vi "final project.vi"() -> ()   [LabVIEW 2014]
uses:
  <vilib>/Utility/file.llb/Read From Spreadsheet File (DBL).vi
  <vilib>/Utility/file.llb/Write To Spreadsheet File (DBL).vi
panel:
  out "發電機開啟":bool
  out "馬達所需能量(W)":dbl(graph)
  out "電池shut down SOC(%)":dbl
  out "電量SOC變化(%)":dbl
  out "剩餘油量(L)":dbl
  out "電量SOC變化(%)":dbl(graph)
  out "油量變化":dbl(graph)
  out "電量需求發電機開啟":bool
  in  "路徑模擬初始值設定":T1={"發電機開啟SOC(%)"="50", "發電機關閉SOC(%)"="80", "電池初始SOC(%) "="100", "電池shut down SOC(%) "="20", "油箱容量(L)"="3"}
  out "引擎熱效率(%)":dbl
  out "發電機效率(%)":dbl
  out "發電機功率(kW)":dbl
  out "電池效率(%)":dbl
  out "功率需求發電機開啟":bool
  out "電池容量(kWh)":dbl
  out "電池最大放電C-rate":dbl
  out "馬達驅動器效率(%)":dbl
  out "馬達效率(%)":dbl
  out "馬達輸出轉速(rpm)":dbl(graph)
  out "馬達輸出扭矩(Nm)":dbl(graph)
  out "車輛目前速度(kph)":dbl(graph)
  in  "停止模擬":bool
  out "馬達輸出轉速":dbl
  out "目標路徑WMTC":dbl(graph)
  out "輪胎半徑(mm)":dbl
  in  "模擬路徑":path=path "E:/碩士班/碩二下課堂/虛擬儀控之設計與應用/WMTC1-2.lvm"
  out "傳動效率(%)":dbl
  out "馬達最大轉速(rpm)":dbl
  out "馬達最大扭矩(Nm)":dbl
  out "馬達功率(kW)":dbl
  out "傳動比":dbl
  in  "開始模擬":bool
  in  "動力系統元件規格":T2={"馬達功率(kW)"="8", "馬達最大扭矩(Nm)"="30", "馬達最大轉速(rpm)"="10000", "發電機功率(kW)"="4", "發電機效率(%)"="90", "引擎熱效率(%)"="20", "電池容量(kWh)"="2", "電池效率(%)"="90", "電池最大放電C-rate"="4", "傳動比"="9", "傳動效率(%)"="85", "馬達效率(%)"="90", "MCU效率(%)"="95"}
  in  "車輛參數設定":T3={"車重(kg)"="150", "人重(kg)"="75", "人數"="1", "CdA (m^2)"="0.37", "滾阻係數"="0.0256", "重力加速度(m/s^2)"="9.81", "空氣密度(kg/m^3)"="1.225", "輪胎半徑(mm)"="0.242"}
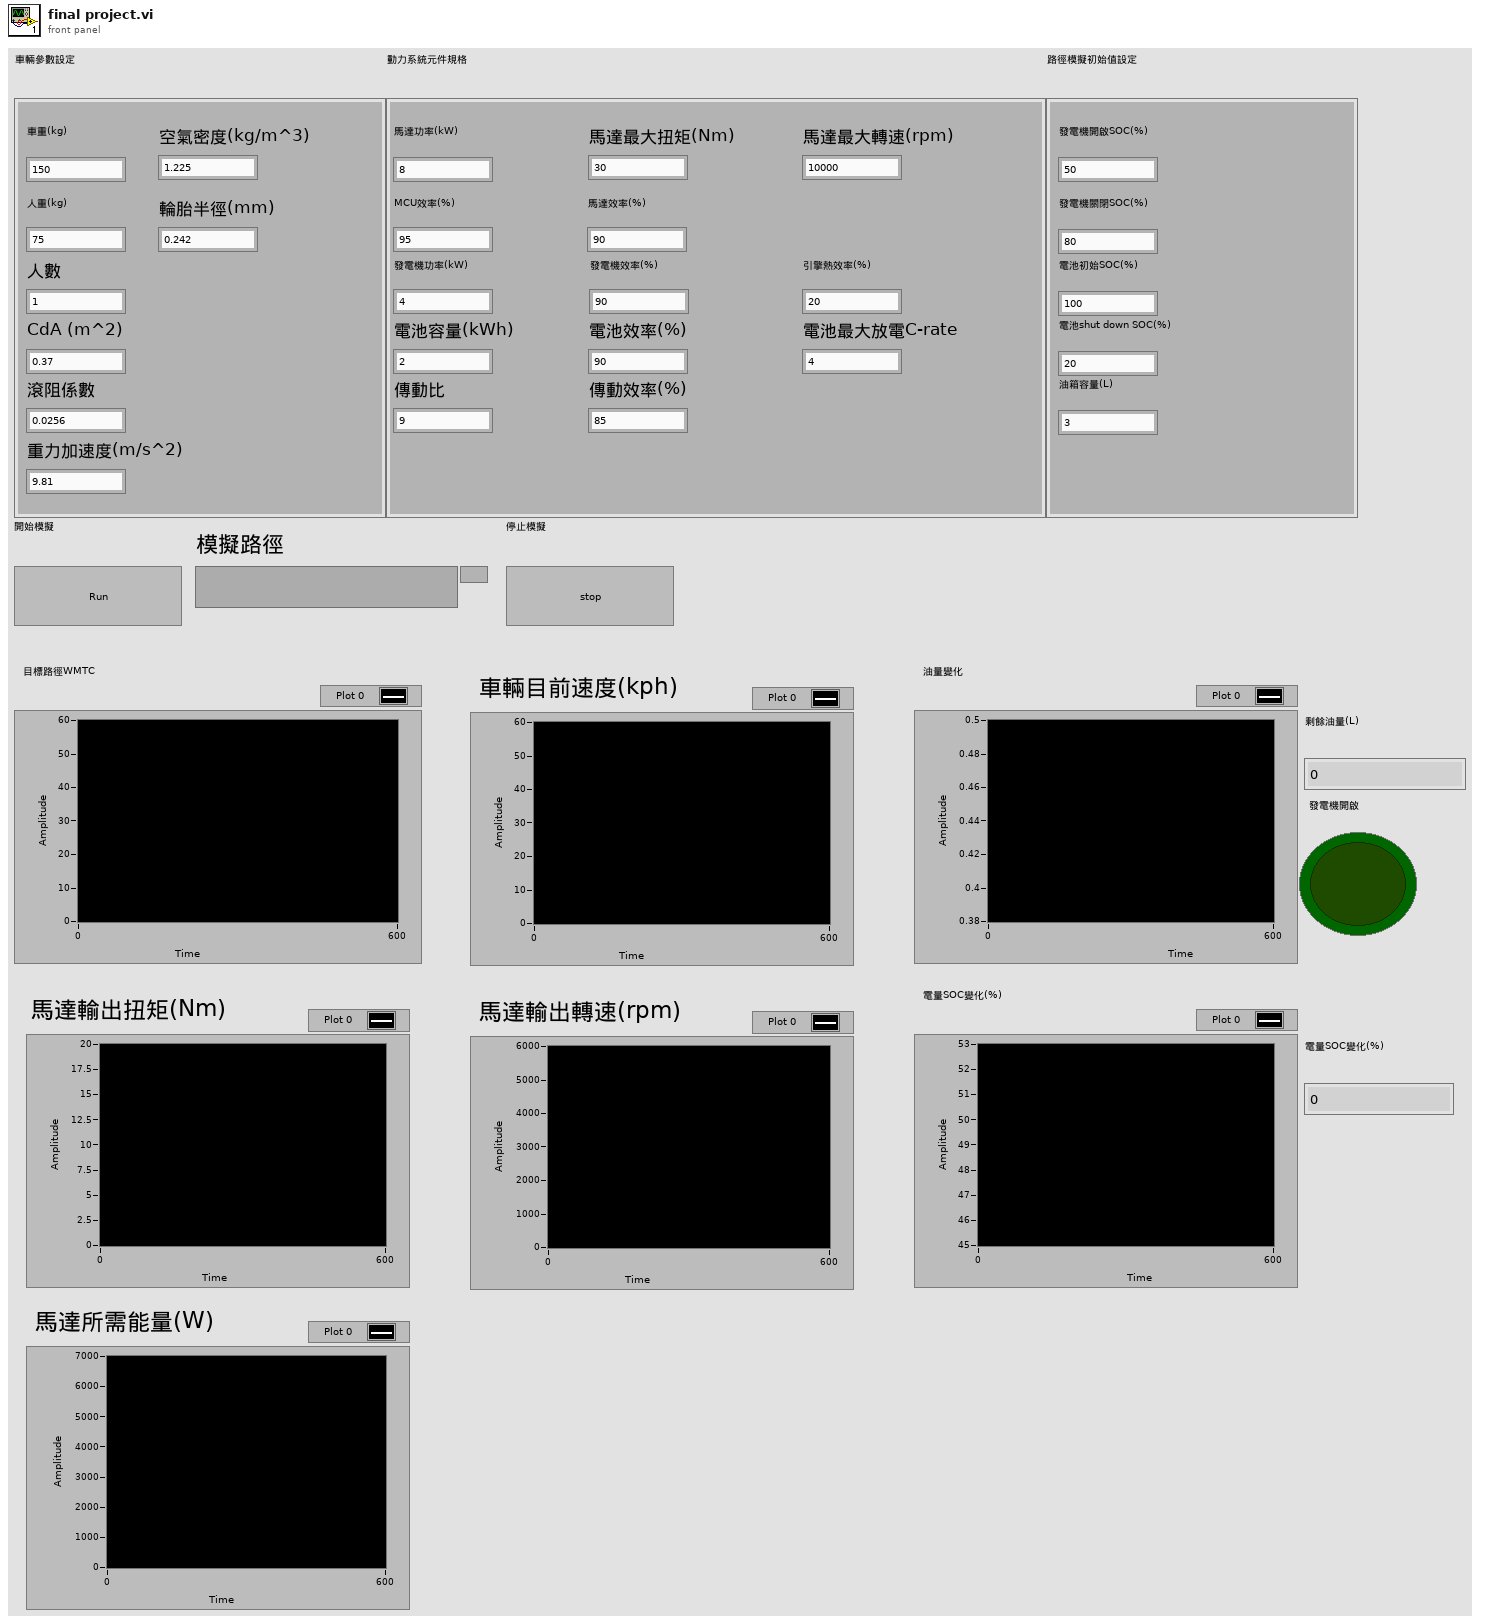
[diagram p1: front panel]
types:
  T1 = cluster{"發電機開啟SOC(%)":string, "發電機關閉SOC(%)":string, "電池初始SOC(%) ":string, "電池shut down SOC(%) ":string, "油箱容量(L)":string}
  T2 = cluster{"馬達功率(kW)":string, "馬達最大扭矩(Nm)":string, "馬達最大轉速(rpm)":string, "發電機功率(kW)":string, "發電機效率(%)":string, "引擎熱效率(%)":string, "電池容量(kWh)":string, "電池效率(%)":string, "電池最大放電C-rate":string, "傳動比":string, "傳動效率(%)":string, "馬達效率(%)":string, "MCU效率(%)":string}
  T3 = cluster{"車重(kg)":string, "人重(kg)":string, "人數":string, "CdA (m^2)":string, "滾阻係數":string, "重力加速度(m/s^2)":string, "空氣密度(kg/m^3)":string, "輪胎半徑(mm)":string}
  T4 = cluster{"馬達功率(kW)":dbl, "馬達最大扭矩(Nm)":dbl, "馬達最大轉速(rpm)":dbl, "發電機功率(kW)":dbl, "發電機效率(%)":dbl, "引擎熱效率(%)":dbl, "電池容量(kWh)":dbl, "電池效率(%)":dbl, "電池最大放電C-rate":dbl, "傳動比":dbl, "傳動效率(%)":dbl, "馬達效率(%)":dbl, "MCU效率(%)":dbl}
  T5 = cluster{"發電機開啟SOC(%)":dbl, "發電機關閉SOC(%)":dbl, "電池初始SOC(%) ":dbl, "電池shut down SOC(%) ":dbl, "油箱容量(L)":dbl}
  T6 = cluster{"車重(kg)":dbl, "人重(kg)":dbl, "人數":dbl, "CdA (m^2)":dbl, "滾阻係數":dbl, "重力加速度(m/s^2)":dbl, "空氣密度(kg/m^3)":dbl, "輪胎半徑(mm)":dbl}
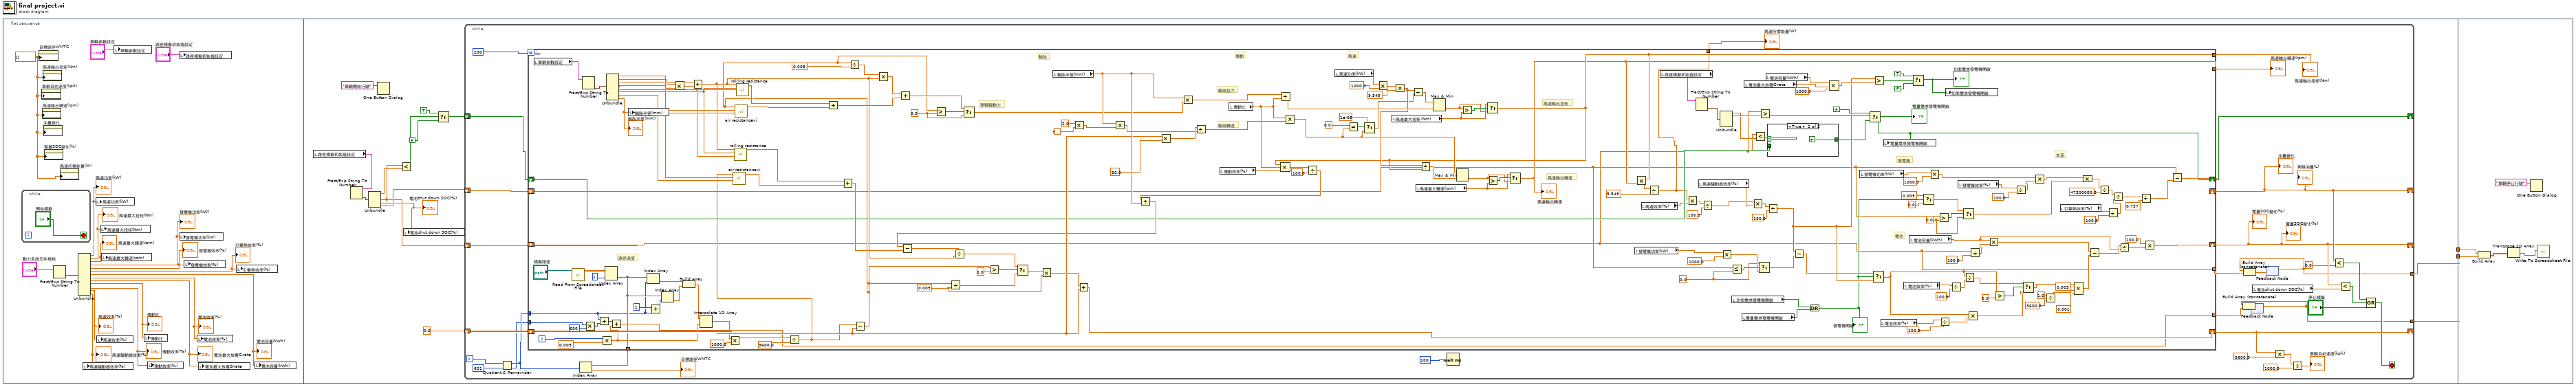
[diagram p0: block diagram]
diagram:
  n1 = flat-sequence {
    tunnel: [w23] -> w2
    tunnel: [w22] -> w1
    tunnel: w2 -> [w259]
    tunnel: w1 -> [w258]
    frame #0 {
      w3 = dbl[] [] ("History Data")
      n2 = while {
        stop <- "開始模擬" stop-if-true
      }
      n3 = property on="目標路徑WMTC" class="WFChart (strict)"("History Data"=w3) -> ()  [unwired: 2 in, 2 out]
      n4 = property on="車輛目前速度(kph)" class="WFChart (strict)"("History Data"=w3) -> ()  [unwired: 2 in, 2 out]
      n5 = property on="馬達輸出轉速(rpm)" class="WFChart (strict)"("History Data"=w3) -> ()  [unwired: 2 in, 2 out]
      n6 = property on="馬達輸出扭矩(Nm)" class="WFChart (strict)"("History Data"=w3) -> ()  [unwired: 2 in, 2 out]
      n7 = property on="油量變化" class="WFChart (strict)"("History Data"=w3) -> ()  [unwired: 2 in, 2 out]
      n8 = property on="電量SOC變化(%)" class="WFChart (strict)"("History Data"=w3) -> ()  [unwired: 2 in, 2 out]
      n9 = Fract/Exp String To Number(string="動力系統元件規格") -> (number=w19:T4)  [unwired: 3 in, 1 out]
      n10 = property on="馬達所需能量(W)" class="WFChart (strict)"("History Data"=w3) -> ()  [unwired: 2 in, 2 out]
      n11 = Unbundle(w19) -> ("馬達功率(kW)"=w17:dbl, "馬達最大扭矩(Nm)"=w16:dbl, "馬達最大轉速(rpm)"=w15:dbl, "發電機功率(kW)"=w7:dbl, "發電機效率(%)"=w6:dbl, "引擎熱效率(%)"=w5:dbl, "電池容量(kWh)"=w9:dbl, "電池效率(%)"=w8:dbl, "電池最大放電C-rate"=w10:dbl, "傳動比"=w18:dbl, "傳動效率(%)"=w14:dbl, "馬達效率(%)"=w12:dbl, "MCU效率(%)"=w11:dbl)
      "傳動比" <- w18
      "馬達功率(kW)" <- w17
      "馬達最大扭矩(Nm)" <- w16
      "馬達最大轉速(rpm)" <- w15
      "傳動效率(%)" <- w14
      "馬達效率(%)" <- w12
      "馬達驅動器效率(%)" <- w11
      "電池最大放電C-rate" <- w10
      "電池容量(kWh)" <- w9
      "電池效率(%)" <- w8
      "發電機功率(kW)" <- w7
      "發電機效率(%)" <- w6
      "引擎熱效率(%)" <- w5
      n12 = local write "馬達驅動器效率(%)"(w11) -> ()
      n13 = local write "馬達功率(kW)"(w17) -> ()
      n14 = local write "馬達效率(%)"(w12) -> ()
      n15 = local write "馬達最大扭矩(Nm)"(w16) -> ()
      n16 = local write "馬達最大轉速(rpm)"(w15) -> ()
      n17 = local write "車輛參數設定"("車輛參數設定") -> ()
      n18 = local write "傳動比"(w18) -> ()
      n19 = local write "傳動效率(%)"(w14) -> ()
      n20 = local write "路徑模擬初始值設定"("路徑模擬初始值設定") -> ()
      n21 = local write "發電機功率(kW)"(w7) -> ()
      n22 = local write "發電機效率(%)"(w6) -> ()
      n23 = local write "電池效率(%)"(w8) -> ()
      n24 = local write "電池最大放電C-rate"(w10) -> ()
      n25 = local write "引擎熱效率(%)"(w5) -> ()
      n26 = local write "電池容量(kWh)"(w9) -> ()
    }
    frame #1 {
      n27 = local read "路徑模擬初始值設定"() -> (w34:T1)
      n28 = Fract/Exp String To Number(string=w34) -> (number=w33:T5)  [unwired: 3 in, 1 out]
      n29 = Unbundle(w33) -> ("發電機開啟SOC(%)"=w30:dbl, "電池初始SOC(%)"=w29:dbl, "電池shut down SOC(%)"=w32:dbl, "油箱容量(L)"=w31:dbl)  [unwired: 1 out]
      "電池shut down SOC(%)" <- w32
      n30 = One Button Dialog(message="車輛開始行駛") -> ()  [unwired: 1 in, 1 out]
      n31 = Less?(x=w29, y=w30) -> (x < y?=w26:bool)
      n32 = local write "電池shut down SOC(%)"(w32) -> ()
      n33 = Select(t=TRUE, s=w26, f=FALSE) -> (s? t:f=w25:bool)
      n34 = while {
        shift-right: [w61] -> _
        shift-left: 0.0 ("y") -> [w69]
        shift-right: [w53] -> _
        shift-left: w31 -> [w55]
        shift-right: [w52] -> _
        shift-left: w29 -> [w54]
        shift-right: [w44] -> _
        shift-left: w25 -> [w45]
        tunnel: [w40] -> w22
        tunnel: [w37] -> w23
        i -> [w66]
        stop <- w48 stop-if-true
        n35 = Quotient & Remainder(x=w66, y=601) -> (x-y*floor(x/y)=w59:i32, floor(x/y)=w36:i32)
        n36 = for {
          N: 200 -> [_]
          shift-right: [w182] -> w61
          shift-left: w69 -> [w186]
          tunnel: w59 -> [w72]
          tunnel: [w83] -> w60
          tunnel: [w174] -> w57
          tunnel: [w173] -> w56
          shift-right: [w132] -> w52
          shift-left: w54 -> [w78]
          shift-right: [w109] -> w53
          shift-left: w55 -> [w96]
          shift-right: [w85] -> w44
          shift-left: w45 -> [w86]
          tunnel: [w79] -> w43
          tunnel: [w78] -> w42 mode=indexing
          tunnel: [w75] -> w39 mode=indexing
          tunnel: w36 -> [w74]
          i -> [w175]
          w87 = 0.0 ("y")
          w98 = 0.0 ("y")
          w188 = 0.005 ("y")
          w201 = 0.0 ("y")
          # "ま篮"
          # "發電機"
          # "電池"
          # "馬達"
          # "輪胎"
          # "傳動"
          # "車輛驅動力"
          # "路徑速度"
          # "馬達輸出轉速"
          # "馬達輸出扭矩"
          # "輪端轉速"
          # "輪端扭力"
          n37 = local read "車輛參數設定"() -> (w217:T3)
          n38 = call-poly <vilib>:"Read From Spreadsheet File.vi"("file path (dialog if empty)"="模擬路徑") -> ("all rows"=w219:dbl[][])  [unwired: 6 in, 4 out]
          n39 = Fract/Exp String To Number(string=w217) -> (number=w218:T6)  [unwired: 3 in, 1 out]
          n40 = Multiply(x=w74, y=600) -> (x*y=w73:i32)
          n41 = Add(x=w72, y=w73) -> (x+y=w71:i32)
          n42 = Multiply(x=w175, y=0.005) -> (x*y=w76:dbl)
          n43 = Index Array(array=w219, index (col)=1 ("index (row)")) -> (element=w83:dbl[])  [unwired: 1 in]
          n44 = Unbundle(w218) -> ("車重(kg)"=w216:dbl, "人重(kg)"=w214:dbl, "人數"=w215:dbl, "CdA (m^2)"=w212:dbl, "滾阻係數"=w211:dbl, "重力加速度(m/s^2)"=w210:dbl, "空氣密度(kg/m^3)"=w209:dbl, "輪胎半徑(mm)"=w208:dbl)
          "輪胎半徑(mm)" <- w208
          n45 = Add(x=w71, y=w76) -> (x+y=w75:dbl)
          n46 = local write "輪胎半徑(mm)"(w208) -> ()
          n47 = Index Array(array=w83, index=w72) -> (element=w178:dbl)
          n48 = Add(x=1, y=w72) -> (x+y=w180:i32)
          n49 = Index Array(array=w83, index=w180) -> (element=w177:dbl)
          n50 = Multiply(x=w214, y=w215) -> (x*y=w213:dbl)
          n51 = Build Array(w178, w177) -> (w176:dbl[])
          n52 = Add(x=w216, y=w213) -> (x+y=w194:dbl)
          n53 = Interpolate 1D Array(1:w76, 2:w176) -> (0:w82:dbl)
          n54 = Multiply(x=w82, y=1000.0) -> (x*y=w185:dbl)
          n55 = call "rolling resistance.vi"("fr"=w211, "g"=w210, "Weight"=w194) -> ("result"=w199:dbl)  [unwired: 8 in]
          n56 = call "rolling resistance.vi"("fr"=w211, "g"=w210, "Weight"=w194) -> ("result"=w251:dbl)  [unwired: 8 in]
          n57 = Divide(x=w185, y=3600.0) -> (x/y=w81:dbl)
          n58 = call "air resistancevi.vi"("air density"=w209, "CdA"=w212, "V^2"=w81) -> ("result"=w198:dbl)  [unwired: 8 in]
          n59 = Add(x=w199, y=w198) -> (x+y=w196:dbl)
          n60 = Subtract(x=w81, y=w186) -> (x-y=w80:dbl)
          n61 = call "air resistancevi.vi"("air density"=w209, "CdA"=w212, "V^2"=w80) -> ("result"=w250:dbl)  [unwired: 8 in]
          n62 = Add(x=w251, y=w250) -> (x+y=w204:dbl)
          n63 = Divide(x=w80, y=0.005) -> (x/y=w206:dbl)
          n64 = Multiply(x=w206, y=w194) -> (x*y=w205:dbl)
          n65 = Add(x=w205, y=w204) -> (x+y=w202:dbl)
          n66 = Greater?(x=w80, y=w201) -> (0:w203:bool)
          n67 = Divide(x=w80, y=w188) -> (x/y=w191:dbl)
          n68 = Select(t=w202, s=w203, f=w201) -> (s? t:f=w200:dbl)
          n69 = Greater?(x=w80, y=0.0) -> (0:w192:bool)
          n70 = local read "輪胎半徑(mm)"() -> (w221:dbl)
          n71 = Multiply(x=2.0, y=3.141592653589793) -> (x*y=w247:dbl)
          n72 = Multiply(x=w221, y=w247) -> (x*y=w244:dbl)
          n73 = Multiply(x=w186, y=60.0) -> (x*y=w245:dbl)
          n74 = Multiply(x=w221, y=w200) -> (x*y=w255:dbl)
          n75 = Divide(x=w245, y=w244) -> (x/y=w254:dbl)
          n76 = local read "傳動效率(%)"() -> (w225:dbl)
          n77 = local read "傳動比"() -> (w226:dbl)
          n78 = Divide(x=w255, y=w226) -> (x/y=w253:dbl)
          n79 = Multiply(x=w226, y=w254) -> (x*y=w252:dbl)
          n80 = local read "馬達功率(kW)"() -> (w243:dbl)
          n81 = Equal?(x=0.0, y=w252) -> (x = y?=w233:bool)
          n82 = Select(t=1e-05, s=w233, f=w252) -> (s? t:f=w231:dbl)
          n83 = Multiply(x=w243, y=1000.0) -> (x*y=w241:dbl)
          n84 = local read "馬達最大扭矩(Nm)"() -> (w237:dbl)
          n85 = Multiply(x=w241, y=9.549) -> (x*y=w235:dbl)
          n86 = Divide(x=w235, y=w231) -> (x/y=w239:dbl)
          n87 = local read "馬達最大轉速(rpm)"() -> (w228:dbl)
          n88 = Max & Min(x=w239, y=w253) -> (min(x,y)=w236:dbl)  [unwired: 1 out]
          n89 = Greater?(x=w236, y=w237) -> (0:w238:bool)
          n90 = Select(t=w237, s=w238, f=w236) -> (s? t:f=w174:dbl)
          n91 = Compound Arithmetic op=MULTIPLY(w174, w226, w225) -> (w224:dbl)
          n92 = Divide(x=w224, y=100.0) -> (x/y=w222:dbl)
          n93 = Divide(x=w222, y=w221) -> (x/y=w197:dbl)
          n94 = Subtract(x=w197, y=w196) -> (x-y=w195:dbl)
          n95 = Divide(x=w195, y=w194) -> (x/y=w190:dbl)
          n96 = Select(t=w190, s=w192, f=w191) -> (s? t:f=w189:dbl)
          n97 = Multiply(x=w189, y=w188) -> (x*y=w187:dbl)
          n98 = Add(x=w187, y=w186) -> (x+y=w182:dbl)
          n99 = Divide(x=w235, y=w174) -> (x/y=w234:dbl)
          n100 = Max & Min(x=w252, y=w234) -> (min(x,y)=w227:dbl)  [unwired: 1 out]
          n101 = Greater?(x=w227, y=w228) -> (0:w229:bool)
          n102 = Select(t=w228, s=w229, f=w227) -> (s? t:f=w173:dbl)
          "馬達輸出轉速" <- w173
          n103 = local read "發電機功率(kW)"() -> (w93:dbl)
          n104 = Multiply(x=w174, y=w173) -> (x*y=w172:dbl)
          n105 = local read "馬達效率(%)"() -> (w170:dbl)
          n106 = Divide(x=w172, y=9.549) -> (x/y=w79:dbl)
          n107 = local read "路徑模擬初始值設定"() -> (w108:T1)
          n108 = Multiply(x=w79, y=w170) -> (x*y=w169:dbl)
          n109 = Fract/Exp String To Number(string=w108) -> (number=w107:T5)  [unwired: 3 in, 1 out]
          n110 = local read "馬達驅動器效率(%)"() -> (w165:dbl)
          n111 = Divide(x=w169, y=100.0) -> (x/y=w164:dbl)
          n112 = Unbundle(w107) -> ("發電機開啟SOC(%)"=w105:dbl, "發電機關閉SOC(%)"=w106:dbl)  [unwired: 3 out]
          n113 = Multiply(x=w93, y=1000.0) -> (x*y=w88:dbl)
          n114 = Less Or Equal?(x=w96, y=w87) -> (x <= y?=w97:bool)
          n115 = local read "功率需求發電機開啟"() -> (w158:bool)
          n116 = local read "電量需求發電機開啟"() -> (w103:bool)
          n117 = local read "電池最大放電C-rate"() -> (w162:dbl)
          n118 = Multiply(x=w164, y=w165) -> (x*y=w166:dbl)
          n119 = Less?(x=w78, y=w105) -> (x < y?=w102:bool)
          n120 = Select(t=w87, s=w97, f=w88) -> (s? t:f=w95:dbl)
          n121 = Greater?(x=w78, y=w106) -> (0:w100:bool)
          n122 = local read "電池容量(kWh)"() -> (w163:dbl)
          n123 = Divide(x=w166, y=100.0) -> (x/y=w131:dbl)
          n124 = case shown="True" w102 {
            tunnel: [w256 TRUE] -> w101
            tunnel: w86 -> [w256 _]
            frame False {
            }
            frame True {
            }
          }
          n125 = Subtract(x=w131, y=w95) -> (x-y=w154:dbl)
          n126 = Or(x=w158, y=w103) -> (x .or. y?=w123:bool)
          "發電機開啟" <- w123
          n127 = Compound Arithmetic op=MULTIPLY(w163, w162, 1000.0 ("value")) -> (w160:dbl)
          n128 = local read "發電機功率(kW)"() -> (w129:dbl)
          n129 = Select(t=FALSE, s=w100, f=w101) -> (s? t:f=w85:bool)
          "電量需求發電機開啟" <- w85
          n130 = Select(t=w154, s=w123, f=w131) -> (s? t:f=w90:dbl)
          n131 = Greater?(x=w131, y=w160) -> (0:w159:bool)
          n132 = local read "電池效率(%)"() -> (w151:dbl)
          n133 = local write "電量需求發電機開啟"(w85) -> ()
          n134 = local read "電池效率(%)"() -> (w92:dbl)
          n135 = local read "電池容量(kWh)"() -> (w135:dbl)
          n136 = Select(t=TRUE, s=w159, f=FALSE) -> (s? t:f=w155:bool)
          "功率需求發電機開啟" <- w155
          n137 = Select(t=0.005, s=w123, f=0.0 ("t")) -> (s? t:f=w120:dbl)
          n138 = Multiply(x=w129, y=1000.0) -> (x*y=w125:dbl)
          n139 = Greater?(x=w96, y=w98) -> (0:w99:bool)
          n140 = Divide(x=w151, y=100.0) -> (x/y=w150:dbl)
          n141 = local write "功率需求發電機開啟"(w155) -> ()
          n142 = Divide(x=w92, y=100.0) -> (x/y=w91:dbl)
          n143 = local read "發電機效率(%)"() -> (w126:dbl)
          n144 = Select(t=w120, s=w99, f=w98) -> (s? t:f=w119:dbl)
          n145 = Divide(x=w90, y=w91) -> (x/y=w89:dbl)
          n146 = Multiply(x=w90, y=w150) -> (x*y=w147:dbl)
          n147 = Divide(x=w78, y=100.0) -> (x/y=w139:dbl)
          n148 = Multiply(x=w135, y=w139) -> (x*y=w138:dbl)
          n149 = Greater?(x=w90, y=0.0) -> (0:w148:bool)
          n150 = Divide(x=w126, y=100.0) -> (x/y=w128:dbl)
          n151 = Select(t=w89, s=w148, f=w147) -> (s? t:f=w146:dbl)
          n152 = Multiply(x=w125, y=w128) -> (x*y=w124:dbl)
          n153 = Divide(x=1.0 ("value"), y=3600.0 ("value")) -> (x/y=w144:dbl)
          n154 = local read "引擎熱效率(%)"() -> (w115:dbl)
          n155 = Compound Arithmetic op=MULTIPLY(w146, 0.005 ("value"), w144, 0.001 ("value")) -> (w137:dbl)
          n156 = Compound Arithmetic op=MULTIPLY(w124, w119) -> (w118:dbl)
          n157 = Subtract(x=w138, y=w137) -> (x-y=w136:dbl)
          n158 = Divide(x=w118, y=47300000.0) -> (x/y=w116:dbl)
          n159 = Divide(x=w115, y=100.0) -> (x/y=w113:dbl)
          n160 = Divide(x=w116, y=w113) -> (x/y=w112:dbl)
          n161 = Divide(x=w136, y=w135) -> (x/y=w134:dbl)
          n162 = Divide(x=w112, y=0.737) -> (x/y=w110:dbl)
          n163 = Multiply(x=100.0, y=w134) -> (x*y=w132:dbl)
          n164 = Subtract(x=w96, y=w110) -> (x-y=w109:dbl)
        }
        "馬達輸出扭矩(Nm)" <- w57
        "馬達輸出轉速(rpm)" <- w56
        "油量變化" <- w53
        "電量SOC變化(%)" <- w52
        "剩餘油量(L)" <- w53
        "電量SOC變化(%)" <- w52
        "馬達所需能量(W)" <- w43
        n165 = Index Array(array=w60, index=w59) -> (element=→"目標路徑WMTC":dbl)
        n166 = Wait (ms)(milliseconds to wait=u32 100) -> ()  [unwired: 1 out]
        n167 = feedback #1() -> (w37:dbl[])  [unwired: 1 in]
        n168 = Build Array (concatenate)(w37, w39) -> (w38:dbl[])
        n169 = feedback-in #1(w38) -> ()
        n170 = local read "電池shut down SOC(%)"() -> (w47:dbl)
        n171 = feedback #2() -> (w40:dbl[])  [unwired: 1 in]
        n172 = Build Array (concatenate)(w40, w42) -> (w41:dbl[])
        n173 = feedback-in #2(w41) -> ()
        n174 = Multiply(x=w61, y=3600.0) -> (x*y=w63:dbl)
        n175 = Divide(x=w63, y=1000.0) -> (x/y=→"車輛目前速度(kph)":dbl)
        n176 = Less?(x=w53, y=0.0 ("x")) -> (x < y?=w51:bool)
        n177 = Less?(x=w52, y=w47) -> (x < y?=w50:bool)
        n178 = Compound Arithmetic op=OR(w51, w50, "停止模擬") -> (w48:bool)
      }
    }
    frame #2 {
      n179 = Build Array(w259, w258) -> (w260:dbl[][])
      n180 = Transpose 2D Array(2D array=w260) -> (transposed array=w261:dbl[][])
      n181 = One Button Dialog(message="車輛停止行駛") -> ()  [unwired: 1 in, 1 out]
      n182 = call-poly <vilib>:"Write To Spreadsheet File.vi"("2D data"=w261) -> ()  [unwired: 7 in, 1 out]
    }
  }
